vi "6.vi"() -> ()   [LabVIEW 2017]
panel:
  out "字符串":string
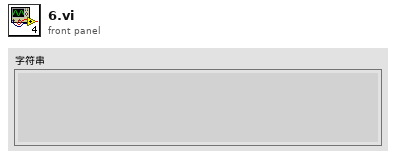
[diagram p1: front panel]
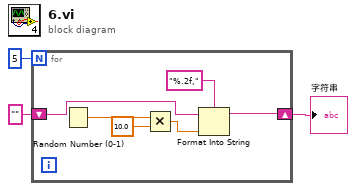
[diagram p0: block diagram]
diagram:
  n1 = for {
    N: 5 -> [_]
    shift-right: [w6] -> w2
    shift-left: "" -> [w5]
    n2 = Random Number (0-1)() -> (number: 0 to 1=w9:dbl)
    n3 = Multiply(x=w9, y=10.0) -> (x*y=w7:dbl)
    n4 = Format Into String(format string="%.2f," ("格式字符串"), initial string=w5, w7) -> (resulting string=w6:string)  [unwired: 1 in, 1 out]
  }
  "字符串" <- w2
